vi "ADCP_Read_and_Update_Packets_From_Serial_Port.vi"(8 "error in (no error)":errorcluster, 11 "ADCP In":refnum<class "ADCP.lvclass">) -> (0 "error out":errorcluster, 1 "Received Packet":u8[](array[numeric]), 2 "Packet Info":T1, 3 "ADCP out":refnum<class "ADCP.lvclass">)   [LabVIEW 2017, in "ADCP.lvclass"]
uses:
  ADCP.lvclass
  ADCP_Packet_Info.ctl
  ADCP.lvclass/ADCP.ctl
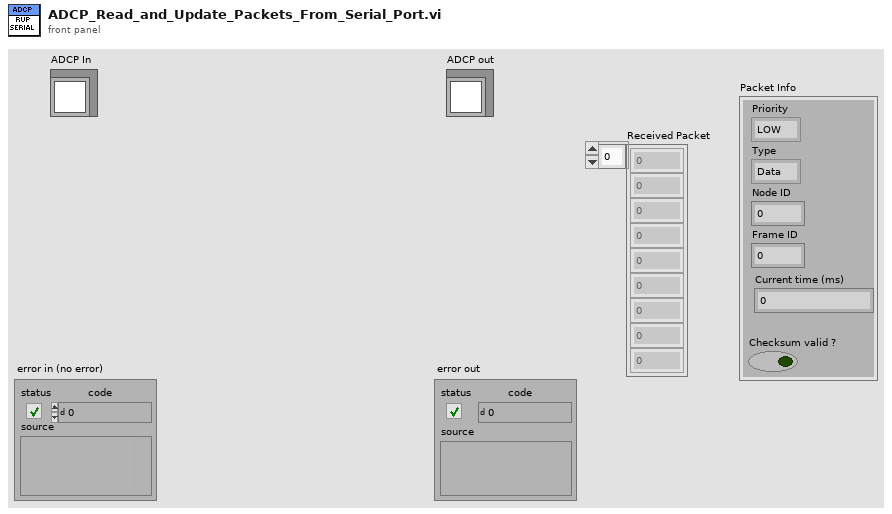
[diagram p1: front panel]
types:
  T1 = typedef "ADCP.lvclass/ADCP_Packet_Info.ctl" = cluster{"Priority":enum16{"LOW", "HIGH"}, "Type":enum16{"Data", "Connection Management", "Remote Request", "Error and status", "INVALID"}, "Node ID":i32, "Frame ID":i32, "Checksum valid ?":bool, "Current time (ms)":u32}
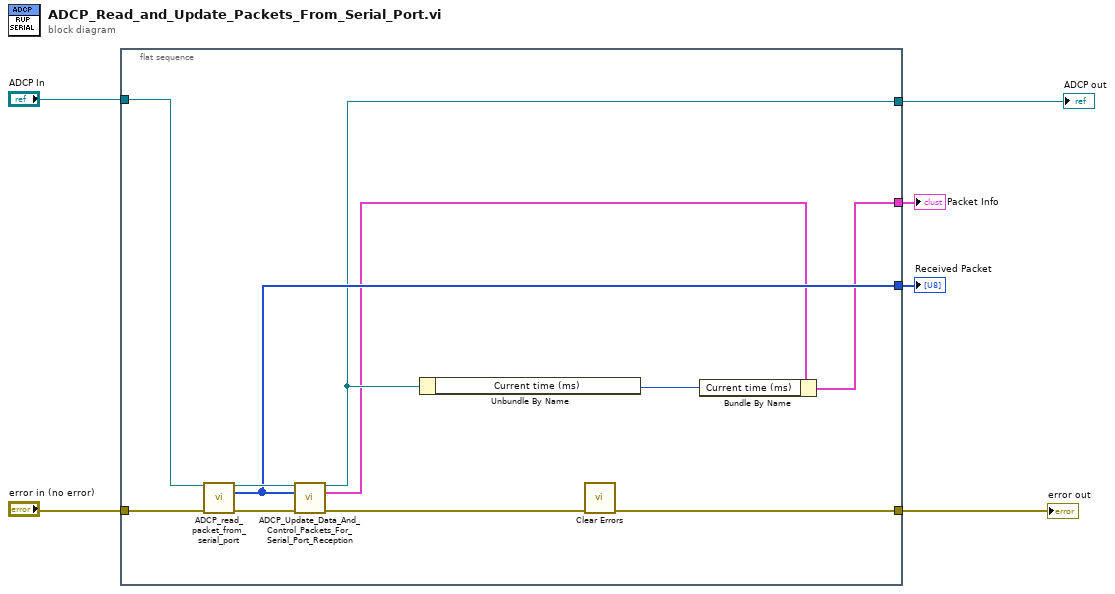
[diagram p0: block diagram]
diagram:
  n1 = flat-sequence {
    tunnel: "error in (no error)" -> [w17]
    tunnel: "ADCP In" -> [w16]
    tunnel: [w12] -> w4
    tunnel: [w7] -> w3
    tunnel: [w9] -> w2
    tunnel: [w13] -> w1
    frame #0 {
      n2 = call "ADCP_read_packet_from_serial_port.vi"("ADCP In"=w16, "error in (no error)"=w17) -> ("ADCP out"=w15:refnum<class "ADCP.lvclass">, "Received Packet"=w13:u8[], "error out"=w14:errorcluster)  [unwired: 6 in, 5 out]
      n3 = call "ADCP_Update_Data_And_Control_Packets_For_Serial_Port_Reception.vi"("ADCP In"=w15, "Processed Packet"=w13, "error in (no error)"=w14) -> ("ADCP out"=w12:refnum<class "ADCP.lvclass">, "Packet Info"=w10:T1, "error out"=w8:errorcluster)  [unwired: 10 in]
      n4 = Unbundle By Name(w12) -> ("Current time (ms)"=w11:u32)
      n5 = call <vilib>:"Clear Errors.vi"("error in (no error)"=w8) -> ("error out"=w7:errorcluster)  [unwired: 5 in, 1 out]
      n6 = Bundle By Name(cluster=w10, "Current time (ms)"=w11) -> (w9:T1)
    }
  }
  "ADCP out" <- w4
  "error out" <- w3
  "Packet Info" <- w2
  "Received Packet" <- w1
